vi "Format Word for CSV.vi"(11 "Word":T1) -> (3 "String Array":string[](array[string]))   [LabVIEW 2020, in "Ballard ARINC 429 Engine.lvlib" / "Implementation.lvlib" / "Word Logging.lvlib" / "CSV Word Logger.lvclass"]
uses:
  CSV Word Logger.lvclass
  Word.ctl
  Word Logging.lvlib
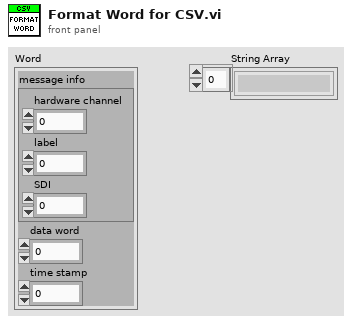
[diagram p1: front panel]
types:
  T1 = typedef "Ballard ARINC 429 Engine.lvlib/Implementation.lvlib/Word Logging.lvlib/Word.ctl" = cluster{"message info":cluster{"hardware channel":u8, "label":u8, "SDI":u8}, "data word":u32, "time stamp":dbl}
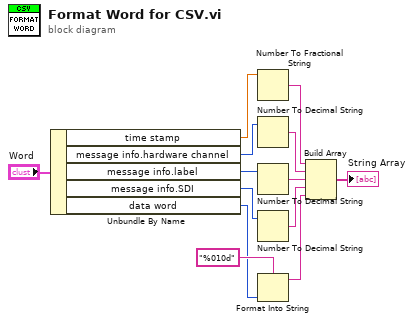
[diagram p0: block diagram]
diagram:
  n1 = Unbundle By Name("Word") -> ("time stamp"=w5:dbl, "message info.hardware channel"=w4:u8, "message info.label"=w3:u8, "message info.SDI"=w2:u8, "data word"=w11:u32)
  n2 = Number To Fractional String(number=w5) -> (F-format string=w9:string)  [unwired: 3 in]
  n3 = Number To Decimal String(number=w4) -> (decimal integer string=w6:string)  [unwired: 1 in]
  n4 = Number To Decimal String(number=w3) -> (decimal integer string=w8:string)  [unwired: 1 in]
  n5 = Number To Decimal String(number=w2) -> (decimal integer string=w7:string)  [unwired: 1 in]
  n6 = Format Into String(format string="%010d", w11) -> (resulting string=w12:string)  [unwired: 2 in, 1 out]
  n7 = Build Array(w9, w6, w8, w7, w12) -> (→"String Array":string[])
